vi "LV FPGA Serial Read Write v1.vi"() -> ()   [LabVIEW 2014]
uses:
  <vilib>/rvi/Emulation/niFpgaGetClockAttributes.vi
  <vilib>/rvi/Emulation/niFpgaSctlEmulationGetInTimedLoop.vi
  <vilib>/rvi/Emulation/niFpgaEmulationReportErrorSimple.vi
  <vilib>/rvi/Emulation/niFpgaProcessEmulError.vi
  Controls/Stop.vi
  <vilib>/rvi/eio/common/nirviEmuTemplateMethod_errors.vi
  <vilib>/rvi/Emulation/niFpgaCriticalErrorInLSC.vi
  <vilib>/rvi/Emulation/niFpgaEmulationIsFPGAContextNoSignature.vi
  <vilib>/rvi/errors/niFpgaSetErrorForExecOnDevCompSimple.vi
  <vilib>/rvi/eio/common/nirviEmuReportErrorAndStop.vi
  <vilib>/rvi/DataTransferAndStorage/Container/Common/niFpgaContainerGetUniqueNameForEmu.vi
  <vilib>/rvi/FIFO/Fifo_Resource/nirvififoEmulationSetSize.vi
  <vilib>/rvi/FIFO/Fifo_Resource/nirviFifoEmulationQueueMgr.vi
  <instcachedir>/0/nirviFifoEmulationQueueMgr_E5CAEC123FF24DC58D834DCA3CDAA9B5.lvgen/nirviFifoEmulationQueueMgr_E5CAEC123FF24DC58D834DCA3CDAA9B5_000.vi
  <vilib>/rvi/FIFO/Fifo_Resource/nirvififoEmulationDetermineInputValidOut.vi
  <vilib>/rvi/FIFO/Fifo_Resource/nirvififoEmulationCreateLock.vi
  <vilib>/rvi/FIFO/Fifo_Resource/nirvififoEmulationObtainLock.vi
  <vilib>/rvi/FIFO/Fifo_Resource/nirvififoEmulationReleaseLock.vi
  <vilib>/rvi/occurrence/nirviWaitOnOccurrenceBase.vi
  <vilib>/rvi/errors/nirviReportUnexpectedCaseInternalError.vi
  <vilib>/rvi/errors/nirviReportUnexpectedCaseInternalError (U32).vi
  <vilib>/eio/EIONode/EIONode.xnode
  <vilib>/rvi/DataTransferAndStorage/Container/XNode/niFpgaContainer.xnode
  <vilib>/rvi/FIFO/Fifo_Resource/nirvififoEmulationWrite.vi
panel:
  out "Read: Transmission Error":bool
  in  "baud rate (9600)":u32=31250
  in  "Invert Polarity?":bool
  in  "stop bits (10: 1 bit)":u16(ring)=10 items=["1.0"=10, "1.5"=15, "2.0"=20]
  in  "parity (0:none)":enum16{"None", "Odd", "Even", "Mark", "Space"}(ring)
  in  "data bits (8)":i32=8 min=5 max=8 step=1
  in  "Receive":refnum<k21>="ConnectorA/DIO10"
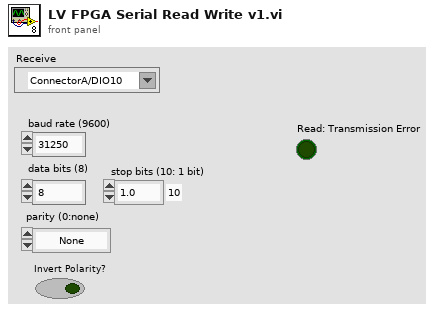
[diagram p1: front panel]
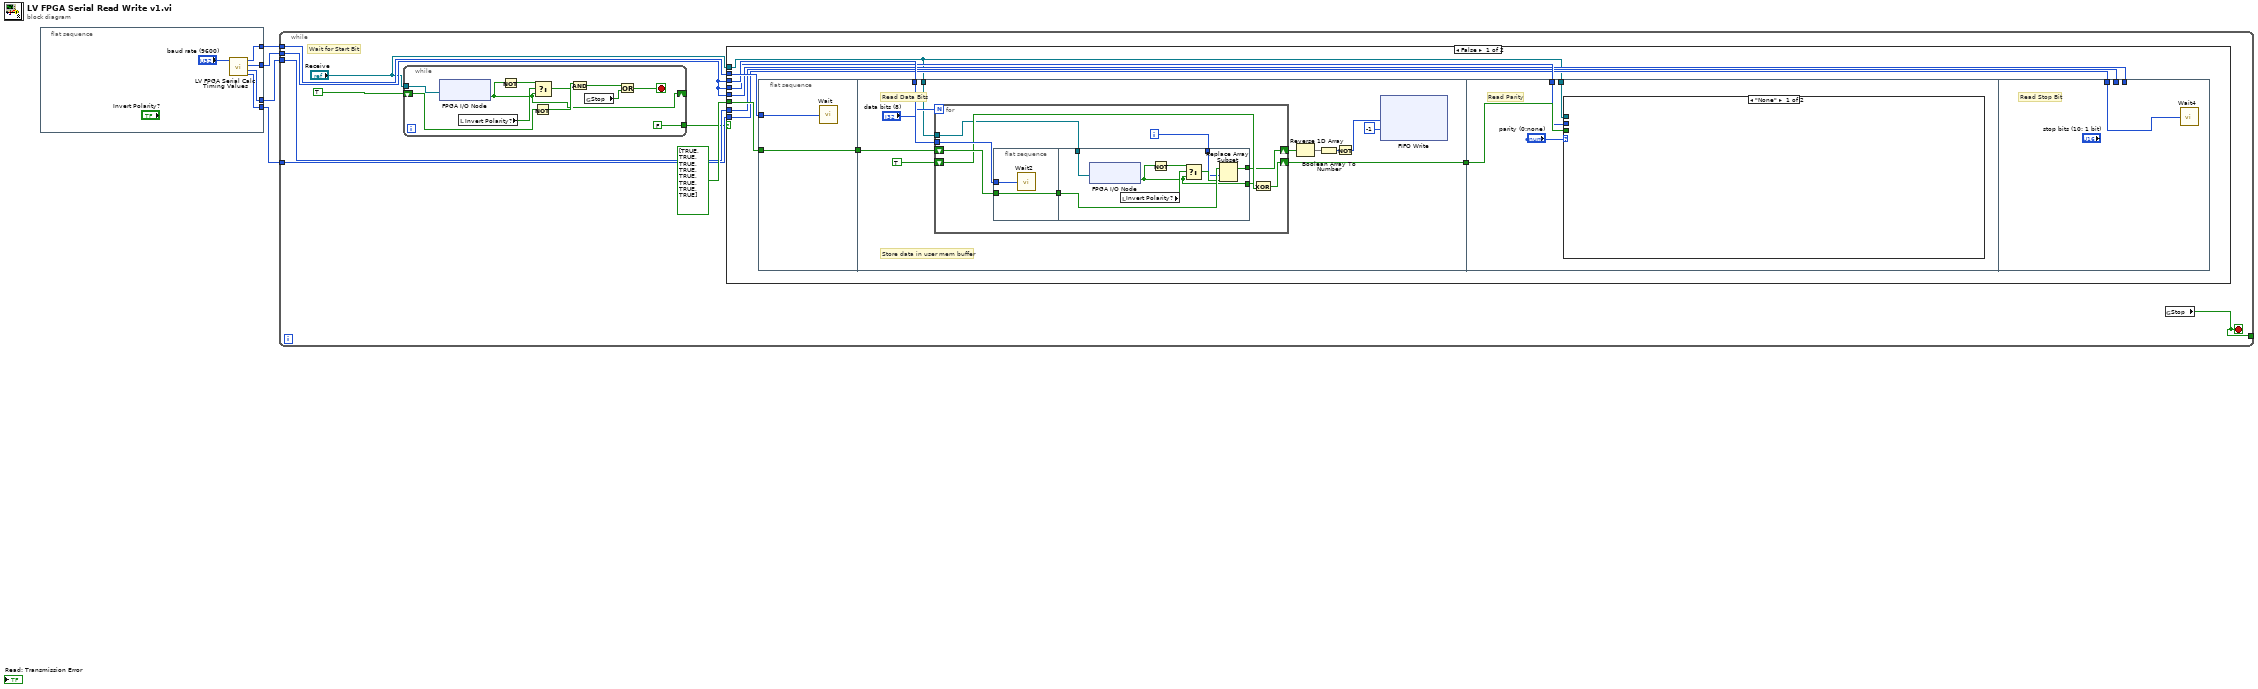
[diagram p0: block diagram]
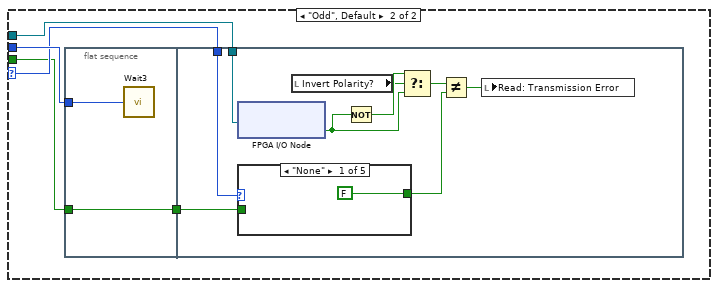
[diagram p2: hidden frame]
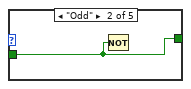
[diagram p3: hidden frame]
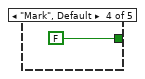
[diagram p5: hidden frame]
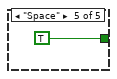
[diagram p6: hidden frame]
diagram:
  n1 = flat-sequence {
    tunnel: [w5] -> w3
    tunnel: [w8] -> w4
    tunnel: [w7] -> w2
    tunnel: [w6] -> w1
    frame #0 {
      n2 = call "LV FPGA Serial Calc Timing Values.vi"("baud rate (1000000)"="baud rate (9600)") -> ("Two Bit"=w6:u32, "One and Half Bit"=w7:u32, "One Bit"=w5:u32, "Half Bit"=w8:u32)  [unwired: 1 in, 2 out]
    }
  }
  n3 = while {
    tunnel: w1 -> [w17]
    tunnel: w2 -> [w16]
    tunnel: w3 -> [w15]
    tunnel: w4 -> [w14]
    tunnel: [w10] -> _
    stop <- w10 stop-if-true
    # "Wait for Start Bit"
    n4 = while {
      tunnel: [FALSE] -> w13
      shift-right: [w20] -> _
      shift-left: TRUE -> [w28]
      tunnel: "Receive" -> [w24]
      stop <- w25 stop-if-true
      n5 = xnode "FPGA I/O Node"("FPGA I/O In"=w24) -> ("I/O Item"=w20:bool)  [unwired: 1 out]
      n6 = local read "Invert Polarity?"() -> (w22:bool)
      n7 = Not(x=w20) -> (.not. x?=w23:bool)
      n8 = Not(x=w28) -> (.not. x?=w27:bool)
      n9 = Select(t=w23, s=w22, f=w20) -> (s? t:f=w21:bool)
      n10 = And(x=w27, y=w21) -> (x .and. y?=w26:bool)
      n11 = global read "Stop.vi" "Stop"() -> (w19:bool)
      n12 = Or(x=w26, y=w19) -> (x .or. y?=w25:bool)
    }
    n13 = case shown="False" w13 {
      tunnel: bool[] [TRUE, TRUE, TRUE, TRUE, TRUE, TRUE, TRUE, TRUE] -> [w38 _]
      tunnel: w14 -> [w37 _]
      tunnel: w15 -> [w36 _]
      tunnel: w15 -> [w35 _]
      tunnel: w15 -> [w34 _]
      tunnel: w16 -> [w33 _]
      tunnel: w17 -> [w32 _]
      tunnel: "Receive" -> [w30 _]
      frame False {
        n14 = flat-sequence {
          tunnel: [w41] -> w39
          tunnel: w38 -> [w41]
          tunnel: w37 -> [w40]
          tunnel: w39 -> [w52]
          tunnel: w36 -> [w51]
          tunnel: [w49] -> w31
          tunnel: w30 -> [w47]
          tunnel: w35 -> [w73]
          tunnel: w31 -> [w75]
          tunnel: w30 -> [w72]
          tunnel: w34 -> [_]
          tunnel: w33 -> [_]
          tunnel: w32 -> [w97]
          frame #0 {
            n15 = call "Wait"("Count(Ticks)"=w40) -> ()  [unwired: 1 out]
          }
          frame #1 {
            # "Store data in user mem buffer"
            # "Read Data Bits"
            n16 = for {
              N: "data bits (8)" -> [_]
              shift-right: [w55] -> w45
              shift-left: w52 -> [w61]
              tunnel: w51 -> [w59]
              shift-right: [w58] -> w49
              shift-left: TRUE -> [w57]
              tunnel: w47 -> [w54]
              i -> [w53]
              n17 = flat-sequence {
                tunnel: w61 -> [w63]
                tunnel: [w63] -> w60
                tunnel: w59 -> [w62]
                tunnel: w60 -> [w71]
                tunnel: [w70] -> w55
                tunnel: [w65] -> w56
                tunnel: w54 -> [w69]
                tunnel: w53 -> [w64]
                frame #0 {
                  n18 = call "Wait2"("Count(Ticks)"=w62) -> ()  [unwired: 1 out]
                }
                frame #1 {
                  n19 = xnode "FPGA I/O Node"("FPGA I/O In"=w69) -> ("I/O Item"=w65:bool)  [unwired: 1 out]
                  n20 = local read "Invert Polarity?"() -> (w68:bool)
                  n21 = Not(x=w65) -> (.not. x?=w67:bool)
                  n22 = Select(t=w67, s=w68, f=w65) -> (s? t:f=w66:bool)
                  n23 = Replace Array Subset(array=w71, new element=w66, index=w64) -> (w70:bool[])
                }
              }
              n24 = Exclusive Or(1:w57, 2:w56) -> (0:w58:bool)
            }
            n25 = Reverse 1D Array(array=w45) -> (reversed array=w44:bool[])
            n26 = Boolean Array To Number(Boolean array=w44) -> (number=w43:u8)
            n27 = Not(x=w43) -> (.not. x?=w42:u8)
            n28 = xnode ("FIFO Write")("Element"=w42, "Timeout"=-1) -> ()  [unwired: 1 in, 2 out]
          }
          frame #2 {
            # "Read Parity"
            n29 = case shown="\"None\"" "parity (0:none)" {
              selector: "parity (0:none)" -> [_ w79]
              tunnel: w75 -> [_ w77]
              tunnel: w73 -> [_ w80]
              tunnel: w72 -> [_ w76]
              frame "None" {
              }
              frame "Odd", Default {
                n30 = flat-sequence {
                  tunnel: w80 -> [w82]
                  tunnel: [w81] -> w78
                  tunnel: w77 -> [w81]
                  tunnel: w79 -> [w91]
                  tunnel: w78 -> [w89]
                  tunnel: w76 -> [w87]
                  frame #0 {
                    n31 = call "Wait3"("Count(Ticks)"=w82) -> ()  [unwired: 1 out]
                  }
                  frame #1 {
                    n32 = xnode "FPGA I/O Node"("FPGA I/O In"=w87) -> ("I/O Item"=w84:bool)  [unwired: 1 out]
                    n33 = case shown="\"None\"" w91 {
                      tunnel: w89 -> [_ w93 w94 _ _]
                      tunnel: [FALSE ("y") w93 w94 FALSE ("y") TRUE ("y")] -> w90
                      frame "None" {
                      }
                      frame "Odd" {
                        n34 = Not(x=w93) -> ()  [unwired: 1 out]
                      }
                      frame "Even" {
                      }
                      frame "Mark", Default {
                      }
                      frame "Space" {
                      }
                    }
                    n35 = local read "Invert Polarity?"() -> (w85:bool)
                    n36 = Not(x=w84) -> (.not. x?=w86:bool)
                    n37 = Select(t=w86, s=w85, f=w84) -> (s? t:f=w83:bool)
                    n38 = Not Equal?(x=w83, y=w90) -> (x != y?=w88:bool)
                    n39 = local write "Read: Transmission Error"(w88) -> ()
                  }
                }
              }
            }
          }
          frame #3 {
            # "Read Stop Bit"
            n40 = call "Wait4"("Count(Ticks)"=w97) -> ()  [unwired: 1 out]
          }
        }
      }
      frame True {
      }
    }
    n41 = global read "Stop.vi" "Stop"() -> (w10:bool)
  }
